vi "Write Signal Name.vi"(8 "error in (no error)":errorcluster, 10 "Signal Name":string, 11 "NF in":refnum<class "NF.lvclass">) -> (0 "error out":errorcluster, 3 "NF out":refnum<class "NF.lvclass">)   [LabVIEW 2018, in "NF.lvlib" / "NF.lvclass"]
uses:
  NF.lvclass
  NF.lvclass/NF.ctl
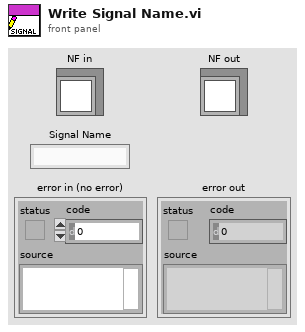
[diagram p1: front panel]
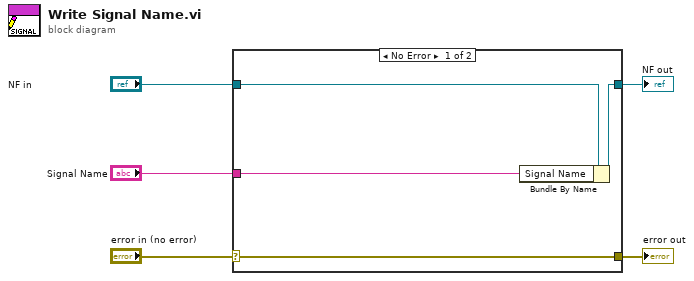
[diagram p0: block diagram]
diagram:
  n1 = case shown="No Error" "error in (no error)" {
    selector: "error in (no error)" -> [w9 w10]
    tunnel: [w9 w10] -> w4
    tunnel: [w7 w11] -> w2
    tunnel: "NF in" -> [w8 w11]
    tunnel: "Signal Name" -> [w6 _]
    frame No Error {
      n2 = Bundle By Name(cluster=w8, "Signal Name"=w6) -> (w7:refnum<class "NF.lvclass">)
    }
    frame Error {
    }
  }
  "error out" <- w4
  "NF out" <- w2
